vi "Data Array to TYpedef.vi"(10 "Module Data Cluster":T4, 11 "first row":dbl[](array[numeric])) -> (2 "Module Data cluster out":T4, 3 "WiBCI 16T Data":T1 {"Reg Map"."ADS2" format="%x"; "Reg Map"."ADS1" format="%x"})   [LabVIEW 2019, in "DemoData Generator.lvlib"]
uses:
  DemoData Generator.lvlib
  Module Data--cluster.ctl
  Acquisition/WiBCI16T_Data.ctl
  Acquisition/WiBCI16T_Status.ctl
  Acquisition/Reg_Map.ctl
  Acquisition/Acquisition.lvlib
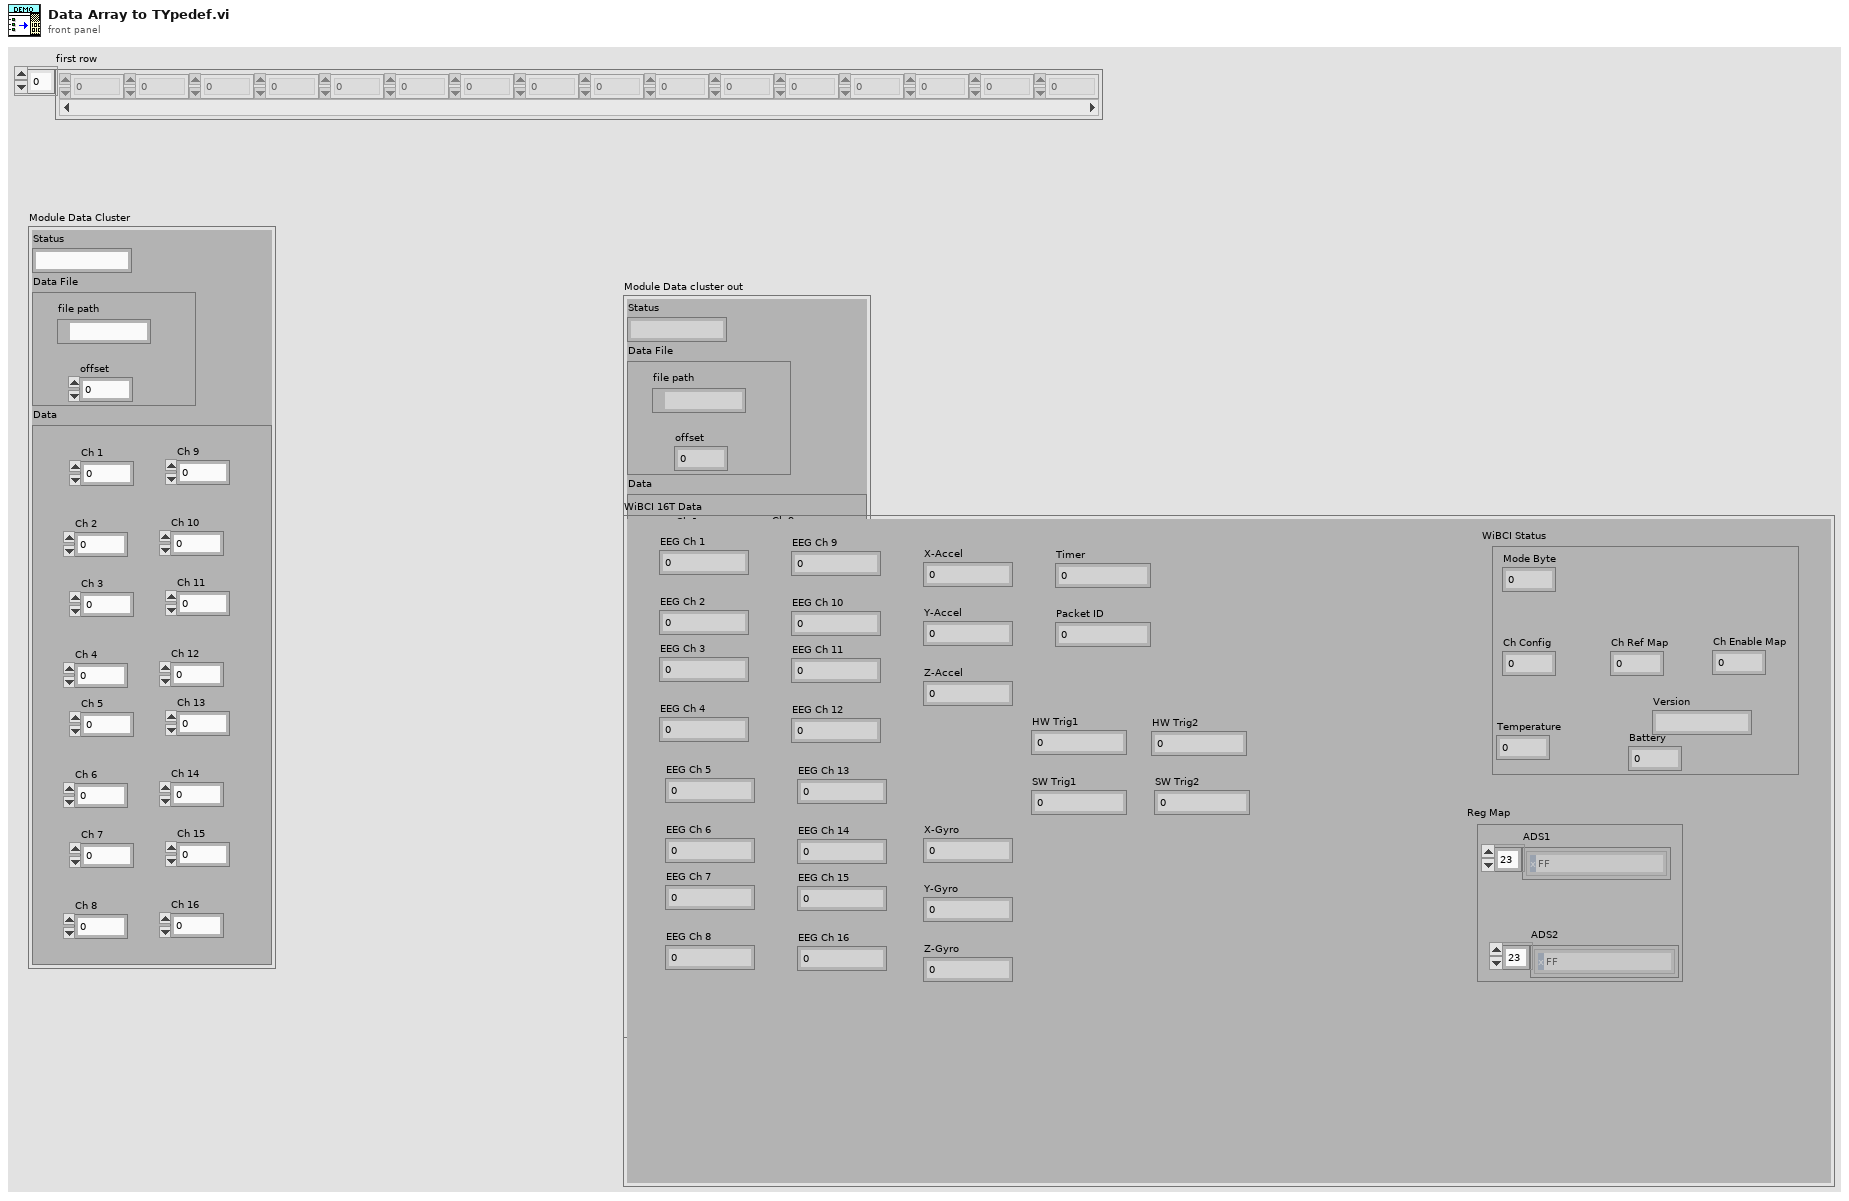
[diagram p1: front panel]
types:
  T1 = typedef "Acquisition.lvlib/WiBCI16T_Data.ctl" = cluster{"EEG Ch 1":dbl, "EEG Ch 2":dbl, "EEG Ch 3":dbl, "EEG Ch 4":dbl, "EEG Ch 5":dbl, "EEG Ch 6":dbl, "EEG Ch 7":dbl, "EEG Ch 8":dbl, "EEG Ch 9":dbl, "EEG Ch 10":dbl, "EEG Ch 11":dbl, "EEG Ch 12":dbl, "EEG Ch 13":dbl, "EEG Ch 14":dbl, "EEG Ch 15":dbl, "EEG Ch 16":dbl, "X-Accel":i16, "Y-Accel":i16, "Z-Accel":i16, "X-Gyro":i16, "Y-Gyro":i16, "Z-Gyro":i16, "Timer":u32, "Packet ID":u32, "HW Trig1":u8, "SW Trig1":i8, "HW Trig2":u8, "SW Trig2":i8, "WiBCI Status":T2, "Reg Map":T3}
  T2 = typedef "Acquisition.lvlib/WiBCI16T_Status.ctl" = cluster{"Mode Byte":u8, "Ch Config":u8, "Ch Ref Map":u16, "Ch Enable Map":u16, "Temperature":sgl, "Battery":u8, "Version":string}
  T3 = typedef "Acquisition.lvlib/Reg_Map.ctl" = cluster{"ADS1":u8[], "ADS2":u8[]}
  T4 = typedef "DemoData Generator.lvlib/Module Data--cluster.ctl" = cluster{"Status":string, "Data File":cluster{"file path":path, "offset":i32}, "Data":cluster{"Ch 1":dbl, "Ch 2":dbl, "Ch 3":dbl, "Ch 4":dbl, "Ch 5":dbl, "Ch 6":dbl, "Ch 7":dbl, "Ch 8":dbl, "Ch 9":dbl, "Ch 10":dbl, "Ch 11":dbl, "Ch 12":dbl, "Ch 13":dbl, "Ch 14":dbl, "Ch 15":dbl, "Ch 16":dbl}}
  T5 = cluster{"Ch 1":dbl, "Ch 2":dbl, "Ch 3":dbl, "Ch 4":dbl, "Ch 5":dbl, "Ch 6":dbl, "Ch 7":dbl, "Ch 8":dbl, "Ch 9":dbl, "Ch 10":dbl, "Ch 11":dbl, "Ch 12":dbl, "Ch 13":dbl, "Ch 14":dbl, "Ch 15":dbl, "Ch 16":dbl}
  T6 = cluster{"[0]":dbl, "[1]":dbl, "[2]":dbl, "[3]":dbl, "[4]":dbl, "[5]":dbl, "[6]":dbl, "[7]":dbl, "[8]":dbl, "[9]":dbl, "[10]":dbl, "[11]":dbl, "[12]":dbl, "[13]":dbl, "[14]":dbl, "[15]":dbl}
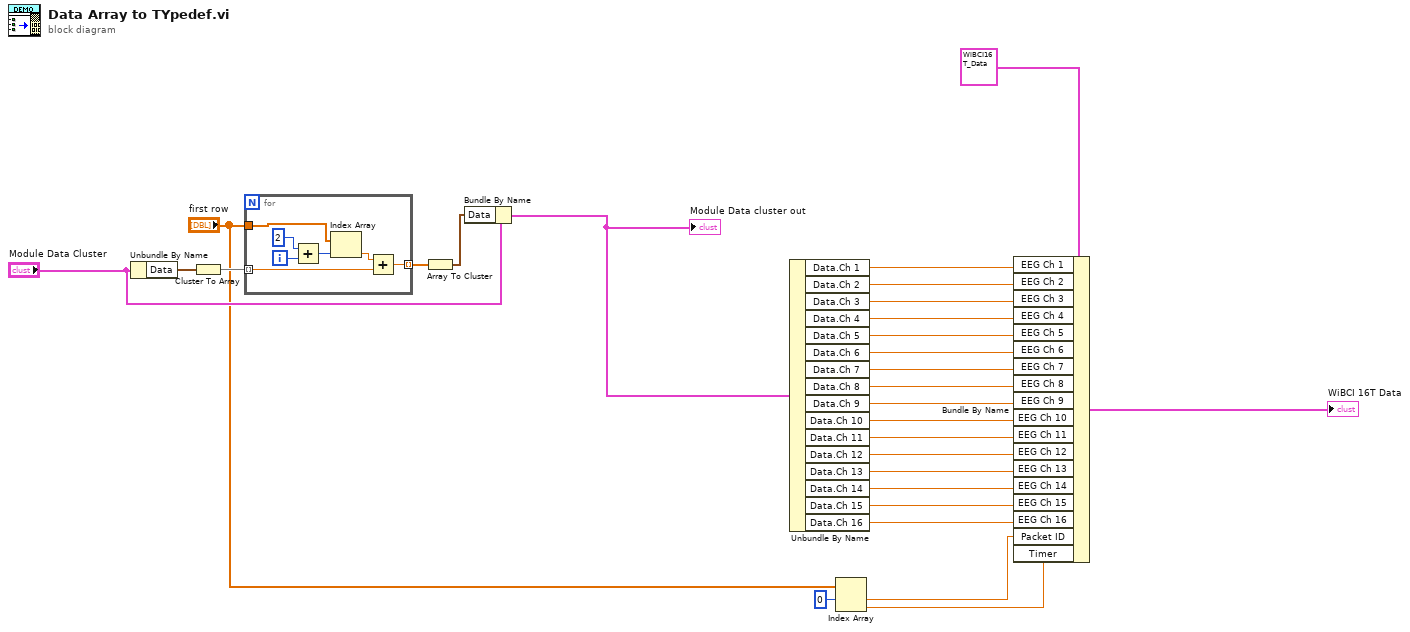
[diagram p0: block diagram]
diagram:
  n1 = Unbundle By Name("Module Data Cluster") -> ("Data"=w28:T5)
  n2 = Cluster To Array(cluster=w28) -> (array=w27:dbl[])
  n3 = for {
    tunnel: "first row" -> [w32]
    tunnel: w27 -> [w30] mode=indexing
    tunnel: [w29] -> w26 mode=indexing
    i -> [w35]
    n4 = Add(x=2, y=w35) -> (x+y=w33:i32)
    n5 = Index Array(array=w32, index=w33) -> (element=w31:dbl)
    n6 = Add(x=w31, y=w30) -> (x+y=w29:dbl)
  }
  n7 = Array To Cluster(array=w26) -> (cluster=w24:T6)
  n8 = Bundle By Name(cluster="Module Data Cluster", "Data"=w24) -> (w22:T4)
  "Module Data cluster out" <- w22
  n9 = Unbundle By Name(w22) -> ("Data.Ch 1"=w17:dbl, "Data.Ch 2"=w16:dbl, "Data.Ch 3"=w15:dbl, "Data.Ch 4"=w14:dbl, "Data.Ch 5"=w13:dbl, "Data.Ch 6"=w12:dbl, "Data.Ch 7"=w11:dbl, "Data.Ch 8"=w10:dbl, "Data.Ch 9"=w9:dbl, "Data.Ch 10"=w8:dbl, "Data.Ch 11"=w7:dbl, "Data.Ch 12"=w6:dbl, "Data.Ch 13"=w5:dbl, "Data.Ch 14"=w4:dbl, "Data.Ch 15"=w3:dbl, "Data.Ch 16"=w2:dbl)
  n10 = Index Array(array="first row", index #1=0 ("index")) -> (element #1=w19:dbl, element #2=w18:dbl)  [unwired: 1 in]
  n11 = Bundle By Name(cluster=T1 {"EEG Ch 1"=0.0, "EEG Ch 2"=0.0, "EEG Ch 3"=0.0, "EEG Ch 4"=0.0, "EEG Ch 5"=0.0, "EEG Ch 6"=0.0, "EEG Ch 7"=0.0, "EEG Ch 8"=0.0, "EEG Ch 9"=0.0, "EEG Ch 10"=0.0, "EEG Ch 11"=0.0, "EEG Ch 12"=0.0, "EEG Ch 13"=0.0, "EEG Ch 14"=0.0, "EEG Ch 15"=0.0, "EEG Ch 16"=0.0, "X-Accel"=0, "Y-Accel"=0, "Z-Accel"=0, "X-Gyro"=0, "Y-Gyro"=0, "Z-Gyro"=0, "Timer"=0, "Packet ID"=0, "HW Trig1"=0, "SW Trig1"=0, "HW Trig2"=0, "SW Trig2"=0, "WiBCI Status"={"Mode Byte"=0, "Ch Config"=0, "Ch Ref Map"=0, "Ch Enable Map"=0, "Temperature"=0.0, "Battery"=0, "Version"=""}, "Reg Map"={"ADS1"=[], "ADS2"=[]}} ("WiBCI16T Data"), "EEG Ch 1"=w17, "EEG Ch 2"=w16, "EEG Ch 3"=w15, "EEG Ch 4"=w14, "EEG Ch 5"=w13, "EEG Ch 6"=w12, "EEG Ch 7"=w11, "EEG Ch 8"=w10, "EEG Ch 9"=w9, "EEG Ch 10"=w8, "EEG Ch 11"=w7, "EEG Ch 12"=w6, "EEG Ch 13"=w5, "EEG Ch 14"=w4, "EEG Ch 15"=w3, "EEG Ch 16"=w2, "Packet ID"=w19, "Timer"=w18) -> (→"WiBCI 16T Data":T1)
